vi "Get IC Array.vi"(5 "target Domain":refnum<class "NI_Domain.lvclass">, 7 "target IC":refnum<class "NI_IC.lvclass">, 8 "error in (no error)":errorcluster, 11 "PDE in":refnum<class "NI_PDE.lvclass">) -> (0 "error out":errorcluster, 2 "IC Array":variant[](array[variant]), 3 "PDE out":refnum<class "NI_PDE.lvclass">)   [LabVIEW 2020, in "NI_PDE.lvlib" / "NI_PDE.lvclass"]
uses:
  <vilib>/gmath/pde.llb/PDEClass/NI_PDE.lvclass
  <vilib>/gmath/pde.llb/ICClass/NI_IC.lvclass
  <vilib>/gmath/pde.llb/DomainClass/NI_Domain.lvclass
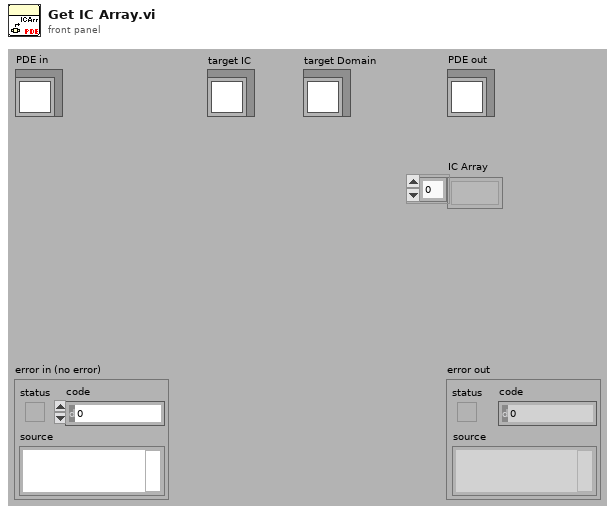
[diagram p1: front panel]
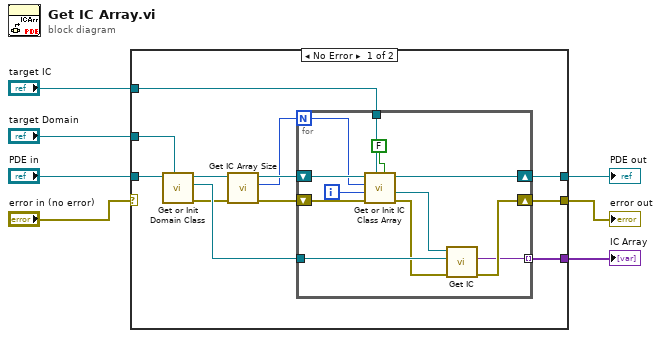
[diagram p0: block diagram]
diagram:
  n1 = case shown="No Error" "error in (no error)" {
    selector: "error in (no error)" -> [_ w33]
    tunnel: "PDE in" -> [w19 w32]
    tunnel: [w15 w32] -> w6
    tunnel: [w14 w33] -> w5
    tunnel: "target IC" -> [w16 _]
    tunnel: "target Domain" -> [w18 _]
    tunnel: [w13 _] -> w1
    frame No Error {
      n2 = call <vilib>:"Get or Init Domain Class.vi"("target Domain"=w18, "PDE out"=w19) -> ("error out"=w11:errorcluster, "Domain out"=w17:refnum<class "NI_Domain.lvclass">, "PDE in"=w12:refnum<class "NI_PDE.lvclass">)  [unwired: 1 in, 6 out]
      n3 = call-dynamic "Get IC Array Size.vi"("error in (no error)"=w11, "PDE in"=w12) -> ("error out"=w9:errorcluster, "# of IC"=w8:i32, "PDE out"=w10:refnum<class "NI_PDE.lvclass">)  [unwired: 7 out]
      n4 = for {
        N: w8 -> [w26]
        shift-right: [w29] -> w15
        shift-left: w10 -> [w30]
        shift-right: [w25] -> w14
        shift-left: w9 -> [w31]
        tunnel: w17 -> [w28]
        tunnel: w16 -> [w24]
        tunnel: [w22] -> w13 mode=indexing
        i -> [w27]
        n5 = call <vilib>:"Get or Init IC Class Array.vi"("type check? (T)"=FALSE, "target IC"=w24, "error in (no error)"=w31, "index"=w27, "# of IC"=w26, "PDE in"=w30) -> ("error out"=w20:errorcluster, "IC out"=w21:refnum<class "NI_IC.lvclass">, "PDE out"=w29:refnum<class "NI_PDE.lvclass">)  [unwired: 3 out]
        n6 = call-dynamic "Get IC.vi"("error in (no error)"=w20, "Domain"=w28, "IC in"=w21) -> ("error out"=w25:errorcluster, "IC"=w22:variant)  [unwired: 7 out]
      }
    }
    frame Error {
    }
  }
  "PDE out" <- w6
  "error out" <- w5
  "IC Array" <- w1
